vi "ArrayStandardDeviation.vi"(10 "Array":dbl[](array[numeric])) -> (1 "StdDev":dbl)   [LabVIEW 2016]
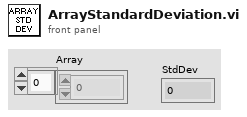
[diagram p1: front panel]
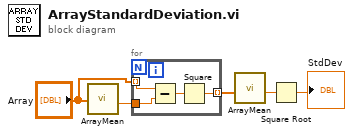
[diagram p0: block diagram]
diagram:
  n1 = call "ArrayMean.vi"("Array"="Array") -> ("Mean"=w3:dbl)  [unwired: 10 in]
  n2 = for {
    tunnel: w3 -> [w9]
    tunnel: "Array" -> [w8] mode=indexing
    tunnel: [w6] -> w1 mode=indexing
    n3 = Subtract(x=w8, y=w9) -> (x-y=w7:dbl)
    n4 = Square(x=w7) -> (x^2=w6:dbl)
  }
  n5 = call "ArrayMean.vi"("Array"=w1) -> ("Mean"=w4:dbl)  [unwired: 10 in]
  n6 = Square Root(x=w4) -> (sqrt(x)=→"StdDev":dbl)
